vi "Topo & GridSpectr_DriftCorrection_zSpec_v15_errorLog.vi"(6 "Internal use":string, 7 "Grid param":T1 {"height (m)" format="%#_6p"; "width (m)" format="%#_6p"; "center Y (m)" format="%#_6p"; "center X (m)" format="%#_6p"}, 8 "Error in (no error)":errorcluster, 9 "Points Y/Index Y":i32, 10 "Points X/Index X":i32, 11 "Method":enum16{"init", "run", "end"}(ring)=enum."end") -> (0 "Error out":errorcluster)   [LabVIEW 2014]
doc: "Example of a measurement VI to be used in the \"Experiments on a Grid\" tool as external VI.\n\nThis example measure the topography and spectroscopy data. The spectroscopy measurements are taken on a subgrid. The data are saved to a sxm and a binary file.\n\n- Nanonis Programming Interface -"
uses:
  <userlib>/Nanonis Prog Interface V5/Scan/Grid/GridPatternGet.vi
  <userlib>/Nanonis Prog Interface V5/Scan/Grid/LinePatternGet.vi
  <userlib>/Nanonis Prog Interface V5/Nanonis Prog Interface.lvlib
panel:
  out "ErrorLog":refnum<file>
  in  "trigger 2 >Hz":sgl format="%#_6p"
  in  "trigger1 < Hz":sgl format="%#_6p"
  out "zFile":refnum<file>
  out "last z adjustment":sgl format="%#_6p"
  in  "during Spec Bias (V)":sgl format="%#_5p"
  in  "type":u16(ring)=1 items=["Line", "Grid"]
  in  "readjust setpoint every":i32=4
  in  "Correct Drift":bool=TRUE
  in  "Email when finished":string="cornelius.krull@monash.edu"
  in  "STS z offset":dbl format="%#_6p"
  out "ETA":timestamp
  out "remaining":dbl format="%<%H:%M:%S>t"
  out "Progress":u8(slide) scale=0.0..100.0 scale format="%#.1g"
  out "total Points":i32
  in  "preSTS delay [ms]":u32=500
  in  "ref Bias":dbl=0.02 format="%#_6p"
  in  "Imaging Bias":dbl=0.02 format="%#_6p"
  in  "max applied Drift Correction":i32=20 min=1 max=100 step=1 format="%.0p"
  in  "Correlate":u16(ring) items=["first Frame", "successive Frames"]
  out "Topo Images taken":i32=14
  in  "Increment":i32=40
  in  "Threshold":i32=2 min=1 step=1
  in  "tip Speed (m/s)":sgl=2e-09 format="%.2p"
  out "X drift":i32
  out "Y drift":i32
  out "Last Drift detected":i32=40
  in  "MaxImagesBack":i32=40
  in  "Channel index (0-23)":u8(ring) items=["Current"=0, "Z (m)"=14]
  in  "File name":string="symmetric_node"
  in  "ref Current":dbl=5e-12 format="%#_6p"
  in  "Imaging Current":dbl=5e-12 format="%#_6p"
  in  "zdrift \nDuration (s)":dbl
  in  "Correct z drift":bool
  out "Status":string="finishing"
  in  "Drift correction Pixels":i32=256 caption="Topo Pixels"
  out "Y Offset":dbl format="%#_6p"
  out "X Offset":dbl format="%#_6p"
  out "Points taken":dbl=14.0
  in  "Drift Correction every":i32=40
  in  "Y subgrid spacing":u16=1
  in  "X subgrid spacing":u16=1
  # "z Spectroscopy"
  # "GRID points"
  # "Increase this if no Drift was detected for \na certain number of images"
  # "%"
  # "time (HH:MM:SS)"
  # "images back"
  # "% of image size"
  # "RUN smart tilt before starting the GRID\nImg Angle = 0\nmove tip to reference point for tip height"
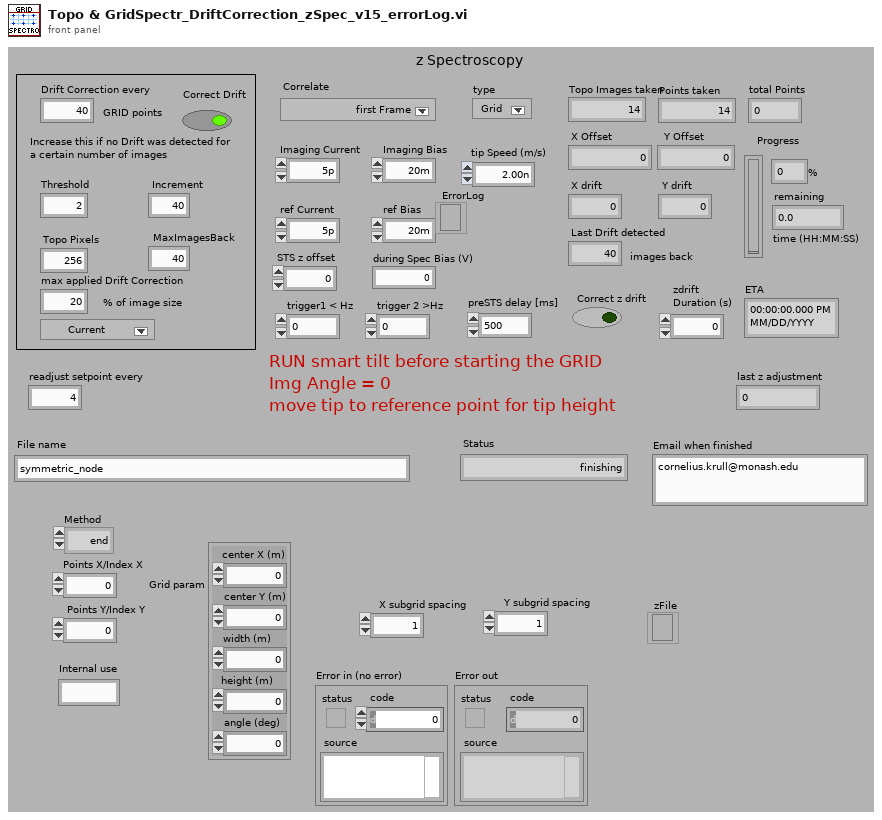
[diagram p1: front panel]
types:
  T1 = cluster{"center X (m)":sgl, "center Y (m)":sgl, "width (m)":sgl, "height (m)":sgl, "angle (deg)":sgl}
  T2 = enum16{"open", "replace", "create", "open or create", "replace or create", "replace or create with confirmation"}
  T3 = cluster{"Z averaging time (s)":sgl, "Z offset (m)":sgl, "Initial settling time (s)":sgl}
  T4 = cluster{"Drift correction Pixels":i32, "Imaging Current":dbl, "STS Current":dbl, "MaxImagesBack":i32, "tip Speed (m/s)":sgl, "Threshold":i32, "Increment":i32, "Correlate":u16, "max applied Drift Correction":i32, "Imaging Bias":dbl, "Move Current":dbl, "Move Bias":dbl, "STS Bias":dbl, "preSTS delay [ms]":u32, "STS z offset":dbl, "Correct Drift":bool, "Lockin ON/OFF":bool}
  T5 = cluster{"center X":sgl, "center Y":sgl, "angle":sgl, "width":sgl, "height":sgl, "# pixels":i32, "# lines":i32}
  T6 = cluster{"Name":string, "Calibration":sgl, "Offset":sgl, "Channel index":i32}[]
  T7 = cluster{"up/down":bool, "time/line":sgl, "start time":timestamp, "end time":timestamp}
  T8 = cluster{"Z averaging time (s)":sgl, "Initial settling time (s)":sgl}
  T9 = cluster{"Max. slew rate (m/s)":sgl, "Settling time (s)":sgl, "Integration time (s)":sgl}
  T10 = cluster{"End settling time (s)":sgl, "Z control time (s)":sgl}
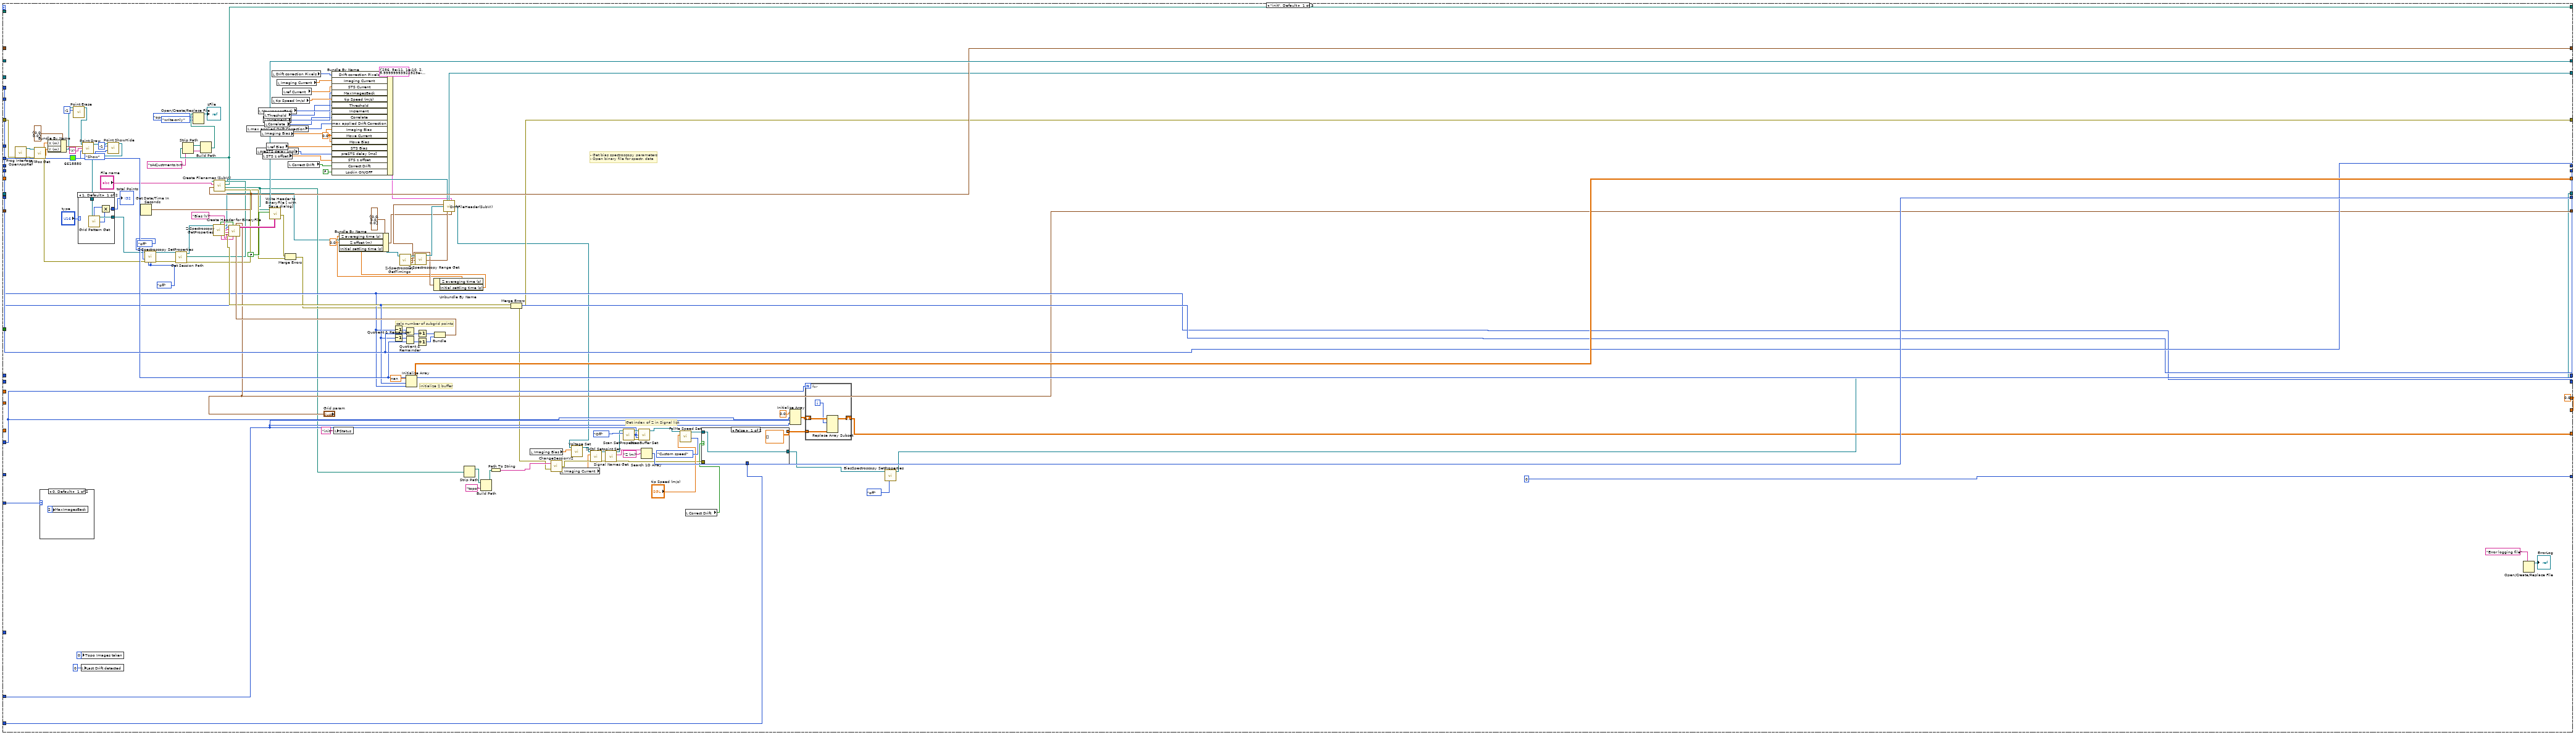
[diagram p2: hidden frame]
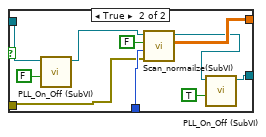
[diagram p3: hidden frame]
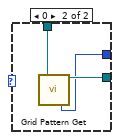
[diagram p4: hidden frame]
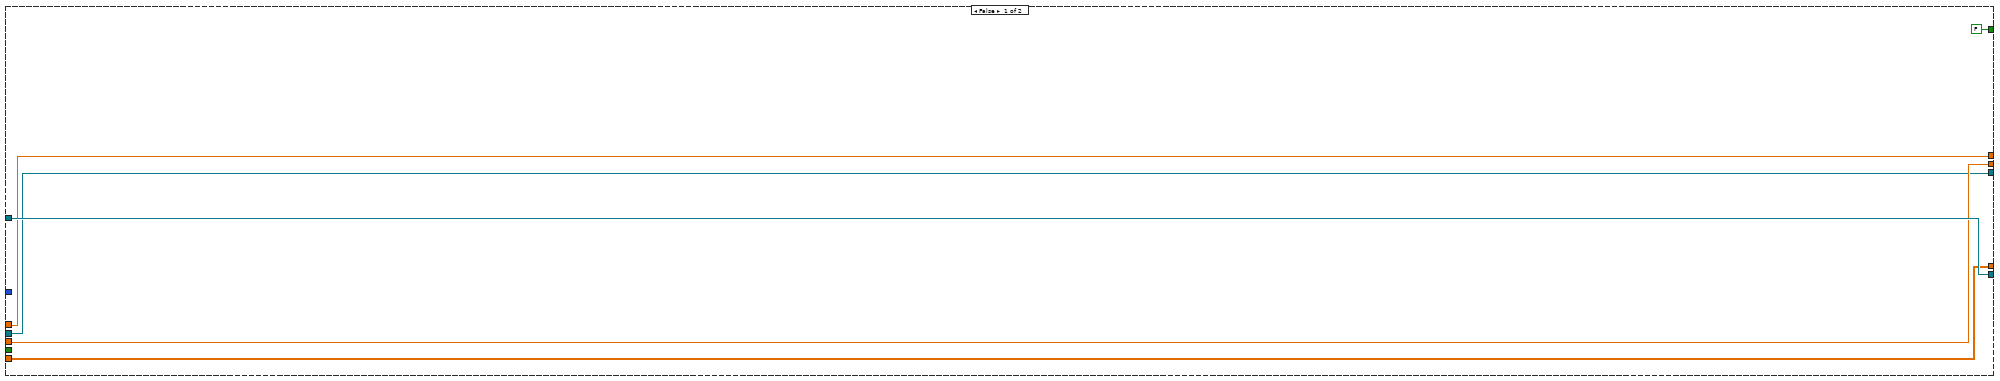
[diagram p9: hidden frame]
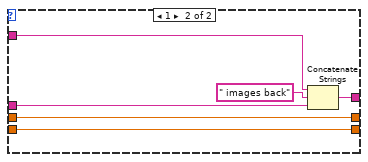
[diagram p10: hidden frame]
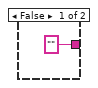
[diagram p12: hidden frame]
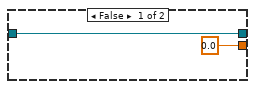
[diagram p13: hidden frame]
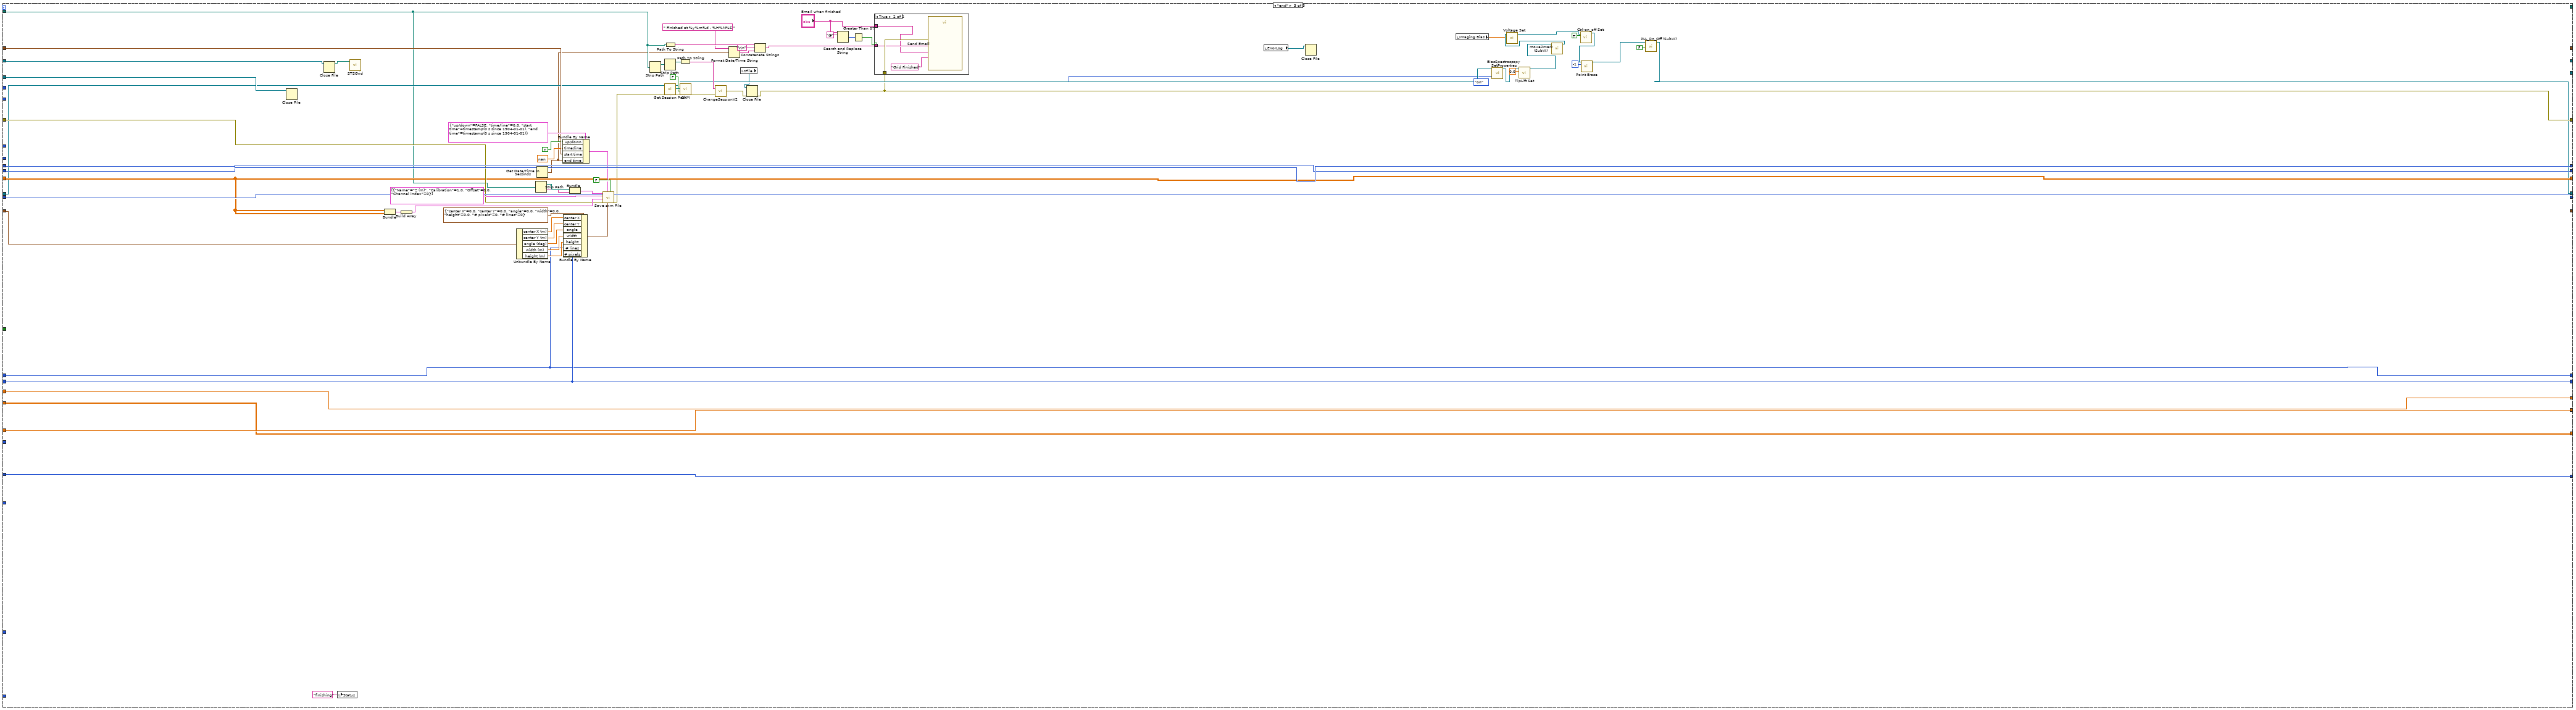
[diagram p15: hidden frame]
diagram:
  # "This string control is required so this VI's connector is compatible with the Nanonis module : \"Experiment on a grid\"."
  # "IMPORTANT : The connector of your own VI must EXACTLY match the connector of this example VI.\n\nThis example VI will do the following:\n- init: Open/Create a sxm (scan data file). Store file path in shift register. Initialize buffer for the topography data. Open binary file and create header.\n- run: Get Z position and write it to topography buffer (from last row to first row of buffer, to make it compatible to Save sxm File function which assumes data starting on the top left corner of image). If grid indices x,y are multiples of the subgrid spacings, start a bias spectroscopy experiment. Write the spectroscopy data to the binary file.\n- end: Write data from topography buffer to file, along with grid dimensions and other known parameters. Close files."
  n1 = while {
    shift-right: [w21] -> _
    shift-left: _ -> [w44]
    shift-right: [w39] -> _
    shift-left: _ -> [w38]
    shift-right: [w36] -> _
    shift-left: _ -> [w37]
    shift-right: [w35] -> _
    shift-left: _ -> [w34]
    shift-right: [w28] -> _
    shift-left: _ -> [w30]
    shift-right: [w29] -> _
    shift-left: _ -> [w31]
    shift-right: [w27] -> _
    shift-left: _ -> [w26]
    shift-right: [w25] -> _
    shift-left: _ -> [w24]
    shift-right: [w23] -> _
    shift-left: _ -> [w22]
    shift-right: [w20] -> _
    shift-left: _ -> [w19]
    shift-right: [w18] -> _
    shift-left: _ -> [w17]
    shift-right: [w16] -> _
    shift-left: _ -> [w9]
    shift-right: [w15] -> _
    shift-left: _ -> [w8]
    shift-right: [w14] -> _
    shift-left: _ -> [w11]
    shift-right: [w13] -> _
    shift-left: _ -> [w10]
    shift-right: [w6] -> _
    shift-left: _ -> [w5]
    stop <- TRUE stop-if-true
    # "> Drift file ref >"
    # "> number of  points  >"
    # "> Ref Frame  >"
    # "> Grid param >"
    # "> start time >"
    # ">Application reference >"
    # "> Y Subgrid spacing >"
    # "> X Subgrid spacing >"
    # "> Z signal index >"
    # "> Binary file ref >"
    # "> Z buffer >"
    # "> sxm file path >"
    n2 = case shown="\"run\"" "Method" {
      tunnel: [w55 w281 _] -> w21
      tunnel: w44 -> [_ w281 w494]
      tunnel: "Error in (no error)" -> [w149 w267 w524]
      tunnel: [w129 w280 w471] -> w42
      tunnel: "Points X/Index X" -> [w161 w275 _]
      tunnel: "Points Y/Index Y" -> [w162 w261 _]
      tunnel: [w185 w278 w513] -> w39
      tunnel: w38 -> [_ w279 w513]
      tunnel: w37 -> [_ w277 w506]
      tunnel: [w177 w276 _] -> w36
      tunnel: [w175 w211 w538] -> w35
      tunnel: w34 -> [_ w211 w538]
      tunnel: "X subgrid spacing" -> [w174 _ _]
      tunnel: "Y subgrid spacing" -> [w173 _ _]
      tunnel: w31 -> [_ w269 w537]
      tunnel: w30 -> [_ w268 w536]
      tunnel: [w174 w269 w537] -> w29
      tunnel: [w173 w268 w536] -> w28
      tunnel: [w114 w254 w469] -> w27
      tunnel: w26 -> [_ w238 w499]
      tunnel: ["Grid param" w264 _] -> w25
      tunnel: w24 -> [_ w264 w523]
      tunnel: [w147 w229 _] -> w23
      tunnel: w22 -> [_ w229 w531]
      tunnel: [w162 w262 w514] -> w20
      tunnel: w19 -> [_ w262 w514]
      tunnel: [w161 w263 w515] -> w18
      tunnel: w17 -> [_ w263 w515]
      tunnel: [w158 w244 w512] -> w16
      tunnel: [w158 w249 w510] -> w15
      tunnel: [w143 w243 w507] -> w14
      tunnel: [0 w227 w511] -> w13
      tunnel: w10 -> [_ w213 w511]
      tunnel: "Drift Correction every" -> [_ w257 _]
      tunnel: w11 -> [_ w248 w507]
      tunnel: w9 -> [_ w255 w512]
      tunnel: w8 -> [_ w241 w510]
      tunnel: "Drift correction Pixels" -> [w142 _ _]
      tunnel: [w110 w246 _] -> w6
      tunnel: w5 -> [_ w247 w508]
      tunnel: "Correct z drift" -> [_ w245 _]
      tunnel: "Channel index (0-23)" -> [w92 w242 _]
      tunnel: "MaxImagesBack" -> [w141 _ _]
      tunnel: "Correlate" -> [w122 _ _]
      frame "init", Default {
        w57 = 0.0 ("Move Current")
        w112 = enum16{"no change", "on", "off"}."off" ("Save dialog")
        w158 = 0.0
        # "- Get bias spectroscopy parameters\n- Open binary file for spectr. data"
        # "initialize Z buffer"
        # "calc number of subgrid points"
        # "Get index of Z in Signal list"
        n3 = call <userlib>:"Prog Interface - OpenAppRef.vi"("Error in (no error)"=w149) -> ("Error out"=w87:errorcluster, "Application reference"=w89:refnum<vi>)  [unwired: 5 in]
        n4 = call <userlib>:"XY-Pos Get.vi"("error in (no error)"=w87, "Application ref in"=w89) -> ("error out"=w88:errorcluster, "Y (m)"=w81:sgl, "X (m)"=w82:sgl, "Application ref out"=w63:refnum<vi>)  [unwired: 5 in]
        n5 = case shown="0, Default" w122 {
          frame 0, Default {
            n6 = local write "MaxImagesBack"(2 ("StepsBack")) -> ()
          }
          frame 1 {
          }
        }
        n7 = Bundle By Name(cluster=cluster{"X (m)":sgl, "Y (m)":sgl} {"X (m)"=0.0, "Y (m)"=0.0} ("Point Coordinates"), "X (m)"=w82, "Y (m)"=w81) -> (w83:cluster{"X (m)":sgl, "Y (m)":sgl})
        n8 = call <userlib>:"Point Erase.vi"("Application ref in"=w63, "Point index (-1=All points)"=-1) -> ("Application ref out"=w62:refnum<vi>)  [unwired: 12 in, 1 out]
        n9 = local write "Topo Images taken"(0 ("Images taken")) -> ()
        n10 = local write "Last Drift detected"(0 ("Last Drift detected")) -> ()
        n11 = call <userlib>:"Point Draw.vi"("Application ref in"=w62, "Point Coordinates"=w83, "Text"="X", "Color"=u32 6618880) -> ("Application ref out"=w67:refnum<vi>)  [unwired: 10 in, 1 out]
        n12 = call <userlib>:"Point ShowHide.vi"("Application ref in"=w67, "Point index (-1=All points)"=-1, "Show/Hide"=enum16{"Show", "Hide"}."Show") -> ("Application ref out"=w66:refnum<vi>)  [unwired: 11 in, 1 out]
        n13 = case shown="1, Default" "type" {
          tunnel: [w202 w205] -> w116
          tunnel: [w199 w203] -> w115
          tunnel: w66 -> [w198 w204]
          frame 1, Default {
            n14 = call-poly <userlib>:"Grid Pattern Get.vi"("Application ref in"=w198) -> ("Points Y"=w200:i32, "Points X"=w201:i32, "Application ref out"=w202:refnum<vi>)  [unwired: 10 in, 6 out]
            n15 = Multiply(x=w200, y=w201) -> (x*y=w199:i32)
          }
          frame 0 {
            n16 = call-poly <userlib>:"Grid Pattern Get.vi"("Application ref in"=w204) -> ("Points"=w203:i32, "Application ref out"=w205:refnum<vi>)  [unwired: 12 in, 5 out]
          }
        }
        "total Points" <- w115
        n17 = Get Date/Time In Seconds() -> (seconds since 1Jan1904=w147:timestamp)
        n18 = call <userlib>:"Z-Spectroscopy SetProperties.vi"("Application ref in"=w116, "Autosave"=enum16{"no change", "on", "off"}."off" ("Autosave (no change)"), "error in (no error)"=w88, "Save dialog"=w112, "Save all sweeps (no change)"=w112) -> ("Application ref out"=w125:refnum<vi>, "error out"=w124:errorcluster)  [unwired: 9 in]
        n19 = call <userlib>:"Get Session Path.vi"("error in (no error)"=w124, "Application ref in"=w125) -> ("error out"=w148:errorcluster, "Session path"=w135:path, "Application ref out"=w126:refnum<vi>)  [unwired: 7 in]
        n20 = call <userlib>:"Z-Spectroscopy GetProperties.vi"("Application ref in"=w126) -> ("Backward sweep"=w181:bool, "Application ref out"=w78:refnum<vi>, "Number of points"=w164:i32, "Channels"=w163:string[], "Parameters"=w179:string[], "Fixed parameters"=w166:string[], "error out"=w178:errorcluster)  [unwired: 7 in, 1 out]
        n21 = call "Create Filenames (SubVI).vi"("error in (no error)"=w148, "seconds since 1Jan1904"=w147, "File name"="File name", "Session path"=w135) -> ("error out"=w138:errorcluster, "binFilePath"=w131:path, "topoFilePath"=w55:path, "Drift File out"=w111:refnum<file>)  [unwired: 4 in]
        n22 = Strip Path(path=w55) -> (stripped path=w54:path)  [unwired: 1 out]
        n23 = Build Path(base path=w54, name or relative path="zAdjustments.txt") -> (appended path=w52:path)
        n24 = Open/Create/Replace File(file path (use dialog)=w52, operation (0:open)=T2."open or create", access (0:read/write)=enum16{"read/write", "read-only", "write-only"}."write-only") -> (refnum out=→"zFile":refnum<file>)  [unwired: 3 in, 2 out]
        n25 = local read "max applied Drift Correction"() -> (w98:i32)
        n26 = local read "preSTS delay [ms]"() -> (w95:u32)
        n27 = local read "MaxImagesBack"() -> (w102:i32)
        n28 = local read "Imaging Bias"() -> (w97:dbl)
        n29 = local read "STS z offset"() -> (w94:dbl)
        n30 = local read "Increment"() -> (w100:i32)
        n31 = local read "Threshold"() -> (w101:i32)
        n32 = local read "Correlate"() -> (w99:u16)
        n33 = local read "ref Bias"() -> (w96:dbl)
        n34 = local read "Drift correction Pixels"() -> (w106:i32)
        n35 = local read "tip Speed (m/s)"() -> (w103:sgl)
        n36 = local read "Imaging Current"() -> (w105:dbl)
        n37 = local read "ref Current"() -> (w104:dbl)
        n38 = local read "Correct Drift"() -> (w93:bool)
        n39 = Bundle By Name(cluster=T4 {"Drift correction Pixels"=256, "Imaging Current"=5e-11, "STS Current"=1e-10, "MaxImagesBack"=2, "tip Speed (m/s)"=1e-08, "Threshold"=2, "Increment"=64, "Correlate"=0, "max applied Drift Correction"=20, "Imaging Bias"=-0.02, "Move Current"=1.5e-11, "Move Bias"=-0.02, "STS Bias"=0.1, "preSTS delay [ms]"=1000, "STS z offset"=-1.7e-10, "Correct Drift"=TRUE, "Lockin ON/OFF"=TRUE} ("Drift Correction"), "Drift correction Pixels"=w106, "Imaging Current"=w105, "STS Current"=w104, "MaxImagesBack"=w102, "tip Speed (m/s)"=w103, "Threshold"=w101, "Increment"=w100, "Correlate"=w99, "max applied Drift Correction"=w98, "Imaging Bias"=w97, "Move Current"=w57, "Move Bias"=w57, "STS Bias"=w96, "preSTS delay [ms]"=w95, "STS z offset"=w94, "Correct Drift"=w93, "Lockin ON/OFF"=FALSE) -> (w108:T4)
        n40 = local write "Status"("init" ("Status")) -> ()
        n41 = Decrement(x=w161) -> (x-1=w172:i32)
        n42 = Decrement(x=w162) -> (x-1=w171:i32)
        n43 = call <userlib>:"Z-Spectroscopy GetTimings.vi"("Application ref in"=w78) -> ("Application ref out"=w79:refnum<vi>, "Initialization"=w74:T8, "Sweep Timing"=w75:T9, "End of Sweep"=w76:T10, "Error out"=w80:errorcluster)  [unwired: 10 in]
        n44 = Quotient & Remainder(x=w172, y=w174) -> (floor(x/y)=w170:i32)  [unwired: 1 out]
        n45 = Quotient & Remainder(x=w171, y=w173) -> (floor(x/y)=w169:i32)  [unwired: 1 out]
        n46 = Initialize Array(sgl nan ("element"), w162, w161) -> (w185:sgl[][])
        n47 = call <userlib>:"Z-Spectroscopy Range Get.vi"("error in (no error)"=w80, "Application ref in"=w79) -> ("Application ref out"=w77:refnum<vi>)  [unwired: 5 in, 3 out]
        n48 = Increment(x=w170) -> (x+1=w168:i32)
        n49 = Increment(x=w169) -> (x+1=w167:i32)
        n50 = Unbundle By Name(w74) -> ("Z averaging time (s)"=w71:sgl, "Initial settling time (s)"=w70:sgl)
        n51 = Bundle By Name(cluster=T3 {"Z averaging time (s)"=0.0, "Z offset (m)"=0.0, "Initial settling time (s)"=0.0} ("Initialization"), "Z averaging time (s)"=w71, "Z offset (m)"=sgl 0.0, "Initial settling time (s)"=w70) -> (w72:T3)
        n52 = Bundle(w168, w167) -> (w180:cluster{i32, i32})  [unwired: 1 in]
        n53 = call <userlib>:"Create Header for BinaryFile.vi"("Grid points"=w180, "Grid param"="Grid param", "Fixed parameters"=w166, "Backward sweep"=w181, "Sweep signal"="Bias (V)" ("Sweep Signal"), "Parameters"=w179, "Channels"=w163, "Points per sweep"=w164) -> ("Header (fixed attributes)"=w183:string[][])  [unwired: 3 in]
        n54 = call <userlib>:"Write Header to BinaryFile [ with Save dialog].vi"("Fixed Attributes"=w183, "Show Dialog? (T)"=FALSE, "Filename"=w131) -> ("Error out"=w139:errorcluster, "File ref"=w177:refnum<file>)  [unwired: 5 in, 2 out]
        n55 = Merge Errors(w139, w138) -> (w140:errorcluster)
        n56 = call "DriftFileHeader(SubVI).vi"("Byte Stream File in"=w111, "Drift Correction"=w108, "End of Sweep"=w76, "Application ref in"=w77, "Sweep Timing"=w75, "Initialization"=w72) -> ("Byte Stream File out"=w110:refnum<file>, "Application ref out"=w109:refnum<vi>)  [unwired: 8 in]
        n57 = Strip Path(path=w131) -> (stripped path=w134:path)  [unwired: 1 out]
        n58 = Build Path(base path=w134, name or relative path="topo") -> (appended path=w132:path)
        n59 = Path To String(path=w132) -> (string=w130:string)
        n60 = Merge Errors(w178, w140) -> (w129:errorcluster)
        n61 = local read "Imaging Bias"() -> (w118:dbl)
        n62 = call "ChangeSessionV2.vi"("error in (no error)"=w129, "Session"=w130) -> ("error out"=w128:errorcluster)
        n63 = local read "Imaging Current"() -> (w117:dbl)
        n64 = call <userlib>:"Voltage Set.vi"("Bias (V)"=w118, "Application ref in"=w109) -> ("Application ref out"=w119:refnum<vi>)  [unwired: 8 in, 1 out]
        n65 = call <userlib>:"Z-Ctrl Setpoint Set.vi"("error in (no error)"=w128, "Z Controller setpoint"=w117, "Application ref in"=w119) -> ("error out"=w150:errorcluster, "Application ref out"=w151:refnum<vi>)  [unwired: 7 in]
        n66 = call <userlib>:"Signal Names Get.vi"("error in (no error)"=w150, "Application ref in"=w151) -> ("error out"=w91:errorcluster, "Signals Names"=w165:string[], "Application ref out"=w154:refnum<vi>)  [unwired: 5 in]
        n67 = call <userlib>:"Scan SetProperties.vi"("Application ref in"=w154, "Continuous scan"=enum16{"No change", "On", "Off"}."Off") -> ("Application ref out"=w156:refnum<vi>, "Error out"=w155:errorcluster)  [unwired: 12 in]
        n68 = call <userlib>:"ScanBuffer Set.vi"("Application ref in"=w156, "Pixels"=w142, "Lines"=w142, "error in (no error)"=w155) -> ("Application ref out"=w120:refnum<vi>)  [unwired: 10 in, 1 out]
        n69 = Search 1D Array(1D array=w165, element="Z (m)") -> (index of element=w175:i32)  [unwired: 1 in]
        n70 = call <userlib>:"FolMe Speed Set.vi"("Speed Setting (Custom)"=enum32{"Scan speed", "Custom speed"}."Custom speed", "Speed (m/s)"="tip Speed (m/s)", "Application ref in"=w120) -> ("Application ref out"=w60:refnum<vi>)  [unwired: 5 in, 1 out]
        n71 = local read "Correct Drift"() -> (w58:bool)
        n72 = case shown="False" w58 {
          tunnel: w92 -> [_ w197]
          tunnel: w91 -> [_ w196]
          tunnel: [dbl[][] [] ("Array") w195] -> w90
          tunnel: w60 -> [w187 w193]
          tunnel: [w187 w188] -> w56
          frame False {
          }
          frame True {
            n73 = call "PLL_On_Off (SubVI).vi"("Output ON/OFF (F=OFF)"=FALSE, "Application in"=w193) -> ("Application out"=w192:refnum<vi>)  [unwired: 8 in, 1 out]
            n74 = call "Scan_normailze(SubVI).vi"("error in (no error)"=w196, "Channel index (0-23)"=w197, "Normalization"=FALSE ("Boolean"), "Application in"=w192) -> ("Array"=w195:dbl[][], "Application out"=w189:refnum<vi>)  [unwired: 5 in, 1 out]
            n75 = call "PLL_On_Off (SubVI).vi"("Output ON/OFF (F=OFF)"=TRUE, "Application in"=w189) -> ("Application out"=w188:refnum<vi>)  [unwired: 8 in, 1 out]
          }
        }
        n76 = Initialize Array(0.0 ("element"), w141, w142, w142) -> (w144:dbl[][][])
        n77 = for {
          N: w141 -> [_]
          tunnel: w90 -> [w209]
          shift-right: [w208] -> w143
          shift-left: w144 -> [w210]
          i -> [w207]
          n78 = Replace Array Subset(array=w210, new element=w209, index (dim 0)=w207) -> (w208:dbl[][][])  [unwired: 2 in]
        }
        n79 = call <userlib>:"BiasSpectroscopy SetProperties.vi"("Application ref in"=w56, "Z-Controller hold (no change)"=enum16{"no change", "on", "off"}."off") -> ("Application ref out"=w114:refnum<vi>)  [unwired: 12 in, 1 out]
        n80 = Open/Create/Replace File(prompt="Error logging file") -> (refnum out=→"ErrorLog":refnum<file>)  [unwired: 5 in, 2 out]
      }
      frame "run" {
        # "shift tip position"
        # "Get Z position"
        # "- get Z position for topography and store it to Z buffer\n- if x,y indices are a multiple of the spacings, take spectroscopy curve and write data to binary file\ndo drift correction if number of STS position was reached"
        n81 = local read "Correct Drift"() -> (w221:bool)
        n82 = Quotient & Remainder(x=w213, y=w257) -> (x-y*floor(x/y)=w258:i32)  [unwired: 1 out]
        n83 = Not Equal To 0?(x=w213) -> (x != 0?=w239:bool)
        n84 = Equal To 0?(x=w258) -> (x = 0?=w256:bool)
        n85 = call <userlib>:"XY-Pos Get.vi"("Wait for newest data (F=False)"=TRUE, "Application ref in"=w238) -> ("Y (m)"=w234:sgl, "X (m)"=w235:sgl, "Application ref out"=w237:refnum<vi>)  [unwired: 5 in, 1 out]
        n86 = Compound Arithmetic op=AND(w239, w256, w221) -> (w240:bool)
        n87 = case shown="True" w240 {
          tunnel: w237 -> [w344 w346]
          tunnel: [w344 w404] -> w218
          tunnel: w248 -> [w341 w400]
          tunnel: [w343 w402] -> w244
          tunnel: [w342 w401] -> w249
          tunnel: w255 -> [w343 w383]
          tunnel: w241 -> [w342 w381]
          tunnel: [w341 w396] -> w243
          tunnel: w247 -> [w340 w407]
          tunnel: [w340 w406] -> w246
          tunnel: w245 -> [_ w403]
          tunnel: w242 -> [_ w387]
          tunnel: [FALSE TRUE] -> w215
          frame False {
          }
          frame True {
            w347 = "Drift Correction" ("Status")
            # "Drift correction \ncompare to the reference image with the previous image \ndx and dy will be applied to the grid coord, \nand the imaging frame will be shifted"
            n88 = Greater Or Equal To 0?(x=w387) -> (x >= 0?=w386:bool)
            n89 = local write "Status"(w347) -> ()
            n90 = case shown="True" w386 {
              frame False {
              }
              frame True {
                n91 = local read "Topo Images taken"() -> (w421:i32)
                n92 = Increment(x=w421) -> (x+1=w420:i32)
                n93 = local write "Topo Images taken"(w420) -> ()
              }
            }
            n94 = local read "Imaging Bias"() -> (w366:dbl)
            n95 = local read "ErrorLog"() -> (w348:refnum<file>)
            n96 = call "ErrorLog (SubVI).vi"("Application ref in"=w346, "Status"=w347, "Byte Stream File in"=w348) -> ("Application ref out"=w345:refnum<vi>)  [unwired: 8 in]
            n97 = call "move2mark (SubVI).vi"("Application in"=w345) -> ("Application out"=w359:refnum<vi>)  [unwired: 10 in]
            n98 = call <userlib>:"Voltage Set.vi"("Bias (V)"=w366, "Application ref in"=w359) -> ("Application ref out"=w367:refnum<vi>)  [unwired: 8 in, 1 out]
            n99 = local read "Imaging Current"() -> (w365:dbl)
            n100 = call <userlib>:"Z-Ctrl Setpoint Set.vi"("Z Controller setpoint"=w365, "Application ref in"=w367) -> ("Application ref out"=w358:refnum<vi>)  [unwired: 8 in, 1 out]
            n101 = call <userlib>:"Ctrl-on_off Set.vi"("Z Controller ON/OFF"=TRUE, "Application ref in"=w358) -> ("Application ref out"=w356:refnum<vi>)  [unwired: 8 in, 1 out]
            n102 = call "PLL_On_Off (SubVI).vi"("Output ON/OFF (F=OFF)"=FALSE, "Application in"=w356) -> ("Application out"=w355:refnum<vi>)  [unwired: 8 in, 1 out]
            n103 = call "Scan_normailze(SubVI).vi"("Channel index (0-23)"=w387, "Normalization"=FALSE ("Boolean"), "Application in"=w355) -> ("Array"=w397:dbl[][], "Application out"=w353:refnum<vi>)  [unwired: 6 in, 1 out]
            n104 = Divide(x="max applied Drift Correction", y=100) -> (x/y=w374:dbl)
            n105 = local read "Drift correction Pixels"() -> (w375:i32)
            n106 = local read "Last Drift detected"() -> (w378:i32)
            n107 = local read "Correlate"() -> (w384:u16)
            n108 = call "PLL_On_Off (SubVI).vi"("Output ON/OFF (F=OFF)"=TRUE, "Application in"=w353) -> ("Application out"=w350:refnum<vi>)  [unwired: 8 in, 1 out]
            n109 = Multiply(x=w374, y=w375) -> (x*y=w376:dbl)
            n110 = call "CorrelImages (SubVI)v2.vi"("last drift detected"=w378, "Correlate"=w384, "Ref Array"=w400, "New Image"=w397) -> ("Y drift"=w372:i32, "X drift"=w369:i32, "Ref Array out"=w396:dbl[][][], "Queue Steps"=w385:i32)  [unwired: 4 in]
            "X drift" <- w369
            "Y drift" <- w372
            "Last Drift detected" <- w385
            n111 = local read "Topo Images taken"() -> (w389:i32)
            n112 = To Long Integer(number=w376) -> (32bit integer=w368:i32)
            n113 = Greater Or Equal?(x=w385, y="Threshold") -> (x >= y?=w391:bool)
            n114 = Greater?(x=w389, y="Threshold") -> (0:w388:bool)
            n115 = call "AbsLimit (SubVI).vi"("in"=w369, "Abslimt"=w368) -> ("Numeric out"=w371:i32)  [unwired: 9 in]
            n116 = call "AbsLimit (SubVI).vi"("in"=w372, "Abslimt"=w368) -> ("Numeric out"=w370:i32)  [unwired: 9 in]
            n117 = And(x=w391, y=w388) -> (x .and. y?=w390:bool)
            n118 = case shown="True" w390 {
              tunnel: ["" w425] -> w392
              frame False {
              }
              frame True {
                n119 = local read "Drift Correction every"() -> (w424:i32)
                n120 = local write "Last Drift detected"(0 ("Last Drift detected")) -> ()
                n121 = Add(x=w424, y="Increment") -> (x+y=w428:i32)
                n122 = local write "Drift Correction every"(w428) -> ()
                n123 = Number To Decimal String(number=w428) -> (decimal integer string=w427:string)  [unwired: 1 in]
                n124 = Concatenate Strings(" Increased DC to every " ("string"), w427) -> (w425:string)
              }
            }
            n125 = local read "Drift correction Pixels"() -> (w394:i32)
            n126 = Number To Decimal String(number=w385) -> (decimal integer string=w399:string)  [unwired: 1 in]
            n127 = case shown="0, Default" w384 {
              tunnel: w399 -> [w408 w419]
              tunnel: [w413 w418] -> w398
              tunnel: w392 -> [w411 w416]
              tunnel: w383 -> [w409 w415]
              tunnel: [w409 w415] -> w382
              tunnel: w381 -> [w410 w414]
              tunnel: [w410 w414] -> w380
              frame 0, Default {
                n128 = Concatenate Strings(w408, "images back , Correlating first frame " ("string"), w411) -> (w413:string)
              }
              frame 1 {
                n129 = Concatenate Strings(w419, " images back" ("string"), w416) -> (w418:string)
              }
            }
            n130 = call "drift_pixel2m (SubVI).vi"("Application in"=w350, "X drift"=w371, "Y drift"=w370, "Drift correction Pixels"=w394) -> ("Application out"=w393:refnum<vi>, "x drift"=w363:sgl, "y drift"=w362:sgl)  [unwired: 2 in, 1 out]
            n131 = local read "type"() -> (w349:u16)
            n132 = call "ShiftFrame (SubVI).vi"("Y shift"=w362, "X shift"=w363, "Application in"=w393) -> ("Application out"=w395:refnum<vi>)  [unwired: 8 in]
            n133 = call "MoveGrid.vi"("type"=w349, "y"=w362, "x"=w363, "Application ref in"=w395) -> ("Application ref out"=w361:refnum<vi>)  [unwired: 6 in, 1 out]
            n134 = call "shift marks (SubVI).vi"("y"=w362, "x"=w363, "Application in"=w361) -> ("Application out"=w360:refnum<vi>)  [unwired: 7 in, 1 out]
            n135 = case shown="True" w403 {
              tunnel: [0.0 ("z drift") w435] -> w405
              tunnel: w360 -> [w430 w434]
              tunnel: [w430 w433] -> w404
              frame False {
              }
              frame True {
                n136 = call "Zdrift_subVi.vi"("Duration"="zdrift \nDuration (s)", "Application in"=w434) -> ("z drift"=w435:dbl, "Application out"=w433:refnum<vi>)  [unwired: 7 in, 1 out]
              }
            }
            n137 = Add(x=w382, y=w363) -> (x+y=w402:dbl)
            n138 = Add(x=w362, y=w380) -> (x+y=w401:dbl)
            n139 = local write "X Offset"(w402) -> ()
            n140 = local write "Y Offset"(w401) -> ()
            n141 = call "Drift Data to file (SubVI).vi"("z drift"=w405, "Comment"=w398, "y Drift"=w401, "X drift"=w402, "Byte Stream File in"=w407) -> ("Byte Stream File out"=w406:refnum<file>)  [unwired: 6 in]
          }
        }
        n142 = Quotient & Remainder(x=w213, y="readjust setpoint every") -> (x-y*floor(x/y)=w214:i32)  [unwired: 1 out]
        n143 = Equal To 0?(x=w213) -> (x = 0?=w212:bool)
        n144 = Equal To 0?(x=w214) -> (x = 0?=w217:bool)
        n145 = Compound Arithmetic op=OR(w212, w215, w217) -> (w216:bool)
        n146 = case shown="True" w216 {
          tunnel: [w282 w303] -> w219
          tunnel: w218 -> [w282 w284]
          tunnel: w211 -> [_ w305]
          frame False {
          }
          frame True {
            w286 = "adjust setpoint" ("Status")
            n147 = local write "Status"(w286) -> ()
            n148 = local read "ErrorLog"() -> (w285:refnum<file>)
            n149 = call "ErrorLog (SubVI).vi"("Application ref in"=w284, "Status"=w286, "Byte Stream File in"=w285) -> ("Application ref out"=w283:refnum<vi>)  [unwired: 8 in]
            n150 = call "move2mark (SubVI).vi"("Application in"=w283) -> ("Application out"=w308:refnum<vi>)  [unwired: 10 in]
            n151 = local read "ref Bias"() -> (w317:dbl)
            n152 = call <userlib>:"Signal Value Get (Animation period) v2.vi"("Wait for newest data (F=False)"=TRUE, "Signal index (0-79)"=w305, "Application ref in"=w308) -> ("Signal value"=w301:sgl, "Application ref out"=w307:refnum<vi>)  [unwired: 5 in, 1 out]
            n153 = local read "ref Current"() -> (w314:dbl)
            n154 = call <userlib>:"Voltage Set.vi"("Bias (V)"=w317, "Application ref in"=w307) -> ("Application ref out"=w315:refnum<vi>)  [unwired: 8 in, 1 out]
            n155 = flat-sequence {
              tunnel: w315 -> [w322]
              tunnel: [w319] -> w313
              tunnel: w314 -> [w321]
              tunnel: w313 -> [w325]
              tunnel: [w325] -> w312
              tunnel: "preSTS delay [ms]" -> [w323]
              tunnel: w312 -> [w330]
              tunnel: [w327] -> w316
              tunnel: [w328] -> w310
              tunnel: w316 -> [w334]
              tunnel: "preSTS delay [ms]" -> [w333]
              tunnel: w310 -> [_]
              tunnel: [w334] -> w309
              tunnel: [w336] -> w304
              tunnel: w309 -> [w337]
              frame #0 {
                n156 = call <userlib>:"Z-Ctrl Setpoint Set.vi"("Z Controller setpoint"=w321, "Application ref in"=w322) -> ("Application ref out"=w320:refnum<vi>)  [unwired: 8 in, 1 out]
                n157 = call <userlib>:"Ctrl-on_off Set.vi"("Z Controller ON/OFF"=TRUE, "Application ref in"=w320) -> ("Application ref out"=w319:refnum<vi>)  [unwired: 8 in, 1 out]
              }
              frame #1 {
                n158 = Greater Than 0?(x=w323) -> (x > 0?=w324:bool)
                n159 = case shown="True" w324 {
                  tunnel: w323 -> [_ w326]
                  frame False {
                  }
                  frame True {
                    n160 = Wait (ms)(milliseconds to wait=w326) -> ()  [unwired: 1 out]
                  }
                }
              }
              frame #2 {
                n161 = local read "STS z offset"() -> (w328:dbl)
                n162 = call <userlib>:"TipLift Set.vi"("TipLift (m)"=w328, "Application ref in"=w330) -> ("Application ref out"=w329:refnum<vi>)  [unwired: 8 in, 1 out]
                n163 = call <userlib>:"Ctrl-on_off Set.vi"("Z Controller ON/OFF"=FALSE, "Application ref in"=w329) -> ("Application ref out"=w327:refnum<vi>)  [unwired: 8 in, 1 out]
              }
              frame #3 {
                n164 = Greater Than 0?(x=w333) -> (x > 0?=w332:bool)
                n165 = case shown="True" w332 {
                  tunnel: w333 -> [_ w335]
                  frame False {
                  }
                  frame True {
                    n166 = Wait (ms)(milliseconds to wait=w335) -> ()  [unwired: 1 out]
                  }
                }
              }
              frame #4 {
                n167 = call <userlib>:"Voltage Set.vi"("Bias (V)"="during Spec Bias (V)", "Application ref in"=w337) -> ("Application ref out"=w336:refnum<vi>)  [unwired: 8 in, 1 out]
              }
            }
            n168 = Get Date/Time In Seconds() -> (seconds since 1Jan1904=w292:timestamp)
            n169 = Get Date/Time String(date format (0)=enum16{"short", "long", "abbreviated"}."short", seconds (now)=w292, want seconds? (F)=TRUE) -> (date string=w296:string, time string=w295:string)
            n170 = local read "zFile"() -> (w299:refnum<file>)
            n171 = Concatenate Strings(w296, w295, "," ("string")) -> (w294:string)
            n172 = call <userlib>:"Signal Value Get (Animation period) v2.vi"("Wait for newest data (F=False)"=TRUE, "Signal index (0-79)"=w305, "Application ref in"=w304) -> ("Signal value"=w300:sgl, "Application ref out"=w303:refnum<vi>)  [unwired: 5 in, 1 out]
            n173 = Subtract(x=w301, y=w300) -> (x-y=w298:sgl)
            "last z adjustment" <- w298
            n174 = Format Into String(format string="%#g", initial string=w294, w298) -> (resulting string=w289:string)  [unwired: 1 in, 1 out]
            n175 = Concatenate Strings(w289, "\r\n") -> (w288:string)
            n176 = Write to Text File(file (use dialog)=w299, text=w288) -> ()  [unwired: 2 in, 3 out]
          }
        }
        n177 = Quotient & Remainder(x=w275, y=w269) -> (x-y*floor(x/y)=w274:i32)  [unwired: 1 out]
        n178 = Quotient & Remainder(x=w261, y=w268) -> (x-y*floor(x/y)=w273:i32)  [unwired: 1 out]
        n179 = Equal To 0?(x=w274) -> (x = 0?=w272:bool)
        n180 = Equal To 0?(x=w273) -> (x = 0?=w271:bool)
        n181 = And(x=w272, y=w271) -> (x .and. y?=w270:bool)
        n182 = Subtract(x=w262, y=w261) -> (x-y=w260:i32)
        n183 = Decrement(x=w260) -> (x-1=w259:i32)
        n184 = Add(x=w235, y=w244) -> (x+y=w251:dbl)
        n185 = Add(x=w234, y=w249) -> (x+y=w250:dbl)
        n186 = call <userlib>:"XY-Pos Set.vi"("Y (m)"=w250, "X (m)"=w251, "Application ref in"=w219) -> ("Application ref out"=w252:refnum<vi>)  [unwired: 5 in, 1 out]
        n187 = call <userlib>:"Signal Value Get (Animation period).vi"("error in (no error)"=w267, "Signal index (0-47)"=w211, "Application ref in"=w252) -> ("error out"=w266:errorcluster, "Signal value"=w265:sgl, "Application ref out"=w253:refnum<vi>)  [unwired: 5 in]
        n188 = Replace Array Subset(array=w279, new element=w265, index (row)=w259, index (col)=w275) -> (w278:sgl[][])
        n189 = case shown="True" w270 {
          tunnel: [w438 w444] -> w280
          tunnel: w277 -> [w439 w465]
          tunnel: [w439 w463] -> w276
          tunnel: w266 -> [w438 w447]
          tunnel: w253 -> [w437 w441]
          tunnel: [w437 w450] -> w254
          tunnel: [w436 w451] -> w227
          tunnel: w213 -> [w436 w452]
          frame False {
            # "Point indices aren't multiple of subgrid spacing\n=> no spectroscopy at this point"
          }
          frame True {
            w443 = "zSpec" ("Status")
            # "remove Bias from data"
            n190 = local read "ErrorLog"() -> (w442:refnum<file>)
            n191 = call "ErrorLog (SubVI).vi"("Application ref in"=w441, "Status"=w443, "Byte Stream File in"=w442) -> ("Application ref out"=w440:refnum<vi>)  [unwired: 8 in]
            n192 = local write "Status"(w443) -> ()
            n193 = call "zSpec_trigger.vi"("Error in (no error)"=w447, "trigger 2"="trigger 2 >Hz", "trigger1"="trigger1 < Hz", "Application ref in"=w440) -> ("Error out"=w446:errorcluster)  [unwired: 5 in, 1 out]
            n194 = call <userlib>:"Z-Spectroscopy Start.vi"("Application ref in"=w440, "Get data (F=False)"=TRUE ("Get Data (F)"), "error in (no error)"=w447) -> ("Application ref out"=w450:refnum<vi>, "Data"=w462:sgl[][], "Parameters"=w461:sgl[], "error out"=w454:errorcluster)  [unwired: 8 in, 1 out]
            n195 = Delete From Array(array=w462, length=1, index (row)=0 ("index")) -> (array with subset deleted=w460:sgl[][])  [unwired: 1 in, 1 out]
            n196 = Write to Binary File(file (use dialog)=w465, data=w461, error in=w454, 5:FALSE ("prepend array or string size? (T)")) -> (refnum out=w464:refnum<file>, error out=w453:errorcluster)  [unwired: 2 in, 1 out]
            n197 = Write to Binary File(file (use dialog)=w464, data=w460, error in=w453, 5:FALSE ("prepend array or string size? (T)")) -> (refnum out=w463:refnum<file>, error out=w445:errorcluster)  [unwired: 2 in, 1 out]
            n198 = Increment(x=w452) -> (x+1=w451:i32)
            n199 = Merge Errors(w446, w445) -> (w444:errorcluster)
          }
        }
        n200 = Get Date/Time In Seconds() -> (seconds since 1Jan1904=w224:timestamp)
        n201 = local read "total Points"() -> (w230:i32)
        n202 = Subtract(x=w224, y=w229) -> (x-y=w228:dbl)
        n203 = Divide(x=w227, y=w230) -> (x/y=w233:dbl)
        n204 = Subtract(x=w230, y=w227) -> (x-y=w225:i32)
        n205 = Divide(x=w228, y=w227) -> (x/y=w226:dbl)
        n206 = Multiply(x=w226, y=w225) -> (x*y=w223:dbl)
        "remaining" <- w223
        n207 = Multiply(x=w233, y=100.0) -> (x*y=→"Progress":dbl)
        n208 = Add(x=w224, y=w223) -> (x+y=→"ETA":timestamp)
      }
      frame "end" {
        n209 = Close File(refnum=w508) -> ()  [unwired: 1 in, 2 out]
        n210 = Close File(refnum=w506) -> (path=w505:path)  [unwired: 1 in, 1 out]
        n211 = local write "Status"("finishing" ("Status")) -> ()
        n212 = call "STSGrid.vi"("Binary Spectroscopy File"=w505) -> ()  [unwired: 11 in]
        n213 = Bundle(w513, w513) -> (w535:cluster{sgl[][], sgl[][]})  [unwired: 1 in]
        n214 = Build Array(w535) -> (w534:cluster{sgl[][], sgl[][]}[])
        n215 = Unbundle By Name(w523) -> ("center X (m)"=w521:sgl, "center Y (m)"=w520:sgl, "angle (deg)"=w519:sgl, "width (m)"=w518:sgl, "height (m)"=w517:sgl)
        n216 = Strip Path(path=w494) -> (stripped path=w527:path, name=w526:string)
        n217 = Get Date/Time In Seconds() -> (seconds since 1Jan1904=w490:timestamp)
        n218 = Bundle By Name(cluster=T7 {"up/down"=FALSE, "time/line"=0.0, "start time"=timestamp(0 s since 1904-01-01), "end time"=timestamp(0 s since 1904-01-01)} ("Scan param"), "up/down"=TRUE, "time/line"=sgl nan ("input 7"), "start time"=w531, "end time"=w490) -> (w530:T7)
        n219 = Bundle By Name(cluster=T5 {"center X"=0.0, "center Y"=0.0, "angle"=0.0, "width"=0.0, "height"=0.0, "# pixels"=0, "# lines"=0} ("Scanfield"), "center X"=w521, "center Y"=w520, "angle"=w519, "width"=w518, "height"=w517, "# lines"=w514, "# pixels"=w515) -> (w516:T5)
        n220 = Bundle("stripped path"=w527, "name"=w526) -> (w525:cluster{"stripped path":path, "name":string})  [unwired: 1 in]
        n221 = call <userlib>:"Save sxm File.vi"("Auto file naming? (T)"=FALSE, "Scanfield"=w516, "Scan param"=w530, "error in (no error)"=w524, "Channels data"=w534, "Channels config"=T6 [{"Name"="Z (m)", "Calibration"=1.0, "Offset"=0.0, "Channel index"=0}], "Filename control"=w525) -> ("error out"=w500:errorcluster)  [unwired: 2 in, 2 out]
        n222 = Strip Path(path=w494) -> (stripped path=w504:path)  [unwired: 1 out]
        n223 = Strip Path(path=w504) -> (stripped path=w503:path)  [unwired: 1 out]
        n224 = call <userlib>:"Get Session Path.vi"("error in (no error)"=w500, "Application ref in"=w499) -> ("error out"=w496:errorcluster, "Session path"=w498:path, "Application ref out"=w483:refnum<vi>)  [unwired: 7 in]
        n225 = Path To String(path=w494) -> (string=w493:string)
        n226 = Path To String(path=w503) -> (string=w501:string)
        n227 = call "SXM.vi"("Path"=w498, "Delete"=FALSE, "error in"=w496) -> ("error out"=w495:errorcluster)  [unwired: 7 in]
        n228 = call "ChangeSessionV2.vi"("error in (no error)"=w495, "Session"=w501) -> ("error out"=w472:errorcluster)
        n229 = Format Date/Time String(time format string (%c)=" Finished at %y%m%d - %H%M%S ", seconds (now)=w490) -> (date/time string=w489:string)  [unwired: 1 in]
        n230 = local read "zFile"() -> (w470:refnum<file>)
        n231 = Close File(refnum=w470, error in=w472) -> (error out=w471:errorcluster)  [unwired: 1 out]
        n232 = Concatenate Strings(w493, "\r\n", w489) -> (w492:string)
        n233 = Search and Replace String(input string="Email when finished", search string="@") -> (number of replacements=w485:i32)  [unwired: 6 in, 3 out]
        n234 = Greater Than 0?(x=w485) -> (x > 0?=w484:bool)
        n235 = case shown="True" w484 {
          tunnel: w471 -> [_ w542]
          tunnel: w492 -> [_ w540]
          tunnel: "Email when finished" -> [_ w539]
          frame False {
          }
          frame True {
            n236 = call "Send Email"("error in"=w542, "Message"=w540, "Subject"="Grid Finished", "Recipients"=w539) -> ()  [unwired: 7 in, 1 out]
          }
        }
        n237 = local read "ErrorLog"() -> (w466:refnum<file>)
        n238 = Close File(refnum=w466) -> ()  [unwired: 1 in, 2 out]
        n239 = local read "Imaging Bias"() -> (w473:dbl)
        n240 = call <userlib>:"BiasSpectroscopy SetProperties.vi"("Application ref in"=w483, "Z-Controller hold (no change)"=enum16{"no change", "on", "off"}."on") -> ("Application ref out"=w481:refnum<vi>)  [unwired: 12 in, 1 out]
        n241 = call <userlib>:"TipLift Set.vi"("TipLift (m)"=sgl 0.0, "Application ref in"=w481) -> ("Application ref out"=w478:refnum<vi>)  [unwired: 8 in, 1 out]
        n242 = call "move2mark (SubVI).vi"("Application in"=w478) -> ("Application out"=w474:refnum<vi>)  [unwired: 10 in]
        n243 = call <userlib>:"Voltage Set.vi"("Bias (V)"=w473, "Application ref in"=w474) -> ("Application ref out"=w475:refnum<vi>)  [unwired: 8 in, 1 out]
        n244 = call <userlib>:"Ctrl-on_off Set.vi"("Z Controller ON/OFF"=TRUE, "Application ref in"=w475) -> ("Application ref out"=w477:refnum<vi>)  [unwired: 8 in, 1 out]
        n245 = call <userlib>:"Point Erase.vi"("Application ref in"=w477, "Point index (-1=All points)"=-1) -> ("Application ref out"=w468:refnum<vi>)  [unwired: 12 in, 1 out]
        n246 = call "PLL_On_Off (SubVI).vi"("Output ON/OFF (F=OFF)"=FALSE, "Application in"=w468) -> ("Application out"=w469:refnum<vi>)  [unwired: 8 in, 1 out]
      }
    }
    "Error out" <- w42
    "Points taken" <- w10
    "X Offset" <- w9
    "Y Offset" <- w8
  }
